vi "Read Key.vi"(8 "Error In":errorcluster, 11 "Tag In":refnum<class "Variable.lvclass">) -> (0 "Error Out":errorcluster, 2 "Key":string, 3 "Tag Out":refnum<class "Variable.lvclass">)   [LabVIEW 2018, in "Toolkit.lvlib" / "Nodes.lvlib" / "Variable.lvclass"]
uses:
  Variable.lvclass
  Variable.lvclass/Variable.ctl
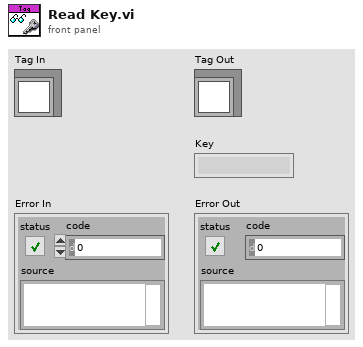
[diagram p1: front panel]
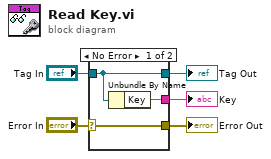
[diagram p0: block diagram]
diagram:
  n1 = case shown="No Error" "Error In" {
    selector: "Error In" -> [w6 w9]
    tunnel: "Tag In" -> [w7 w10]
    tunnel: [w8 _] -> w3
    tunnel: [w7 w10] -> w4
    tunnel: [w6 w9] -> w1
    frame No Error {
      n2 = Unbundle By Name(w7) -> ("Key"=w8:string)
    }
    frame Error {
    }
  }
  "Tag Out" <- w4
  "Key" <- w3
  "Error Out" <- w1
